vi "getState.vi"(8 "error in (no error)":errorcluster, 11 "Electrometer in":refnum<class "Electrometer.lvclass">) -> (0 "error out":errorcluster, 2 "State":T1, 3 "Electrometer out":refnum<class "Electrometer.lvclass">)   [LabVIEW 2016, in "Electrometer.lvclass"]
uses:
  Electrometer.lvclass
  internalState.ctl
  State/State.lvclass
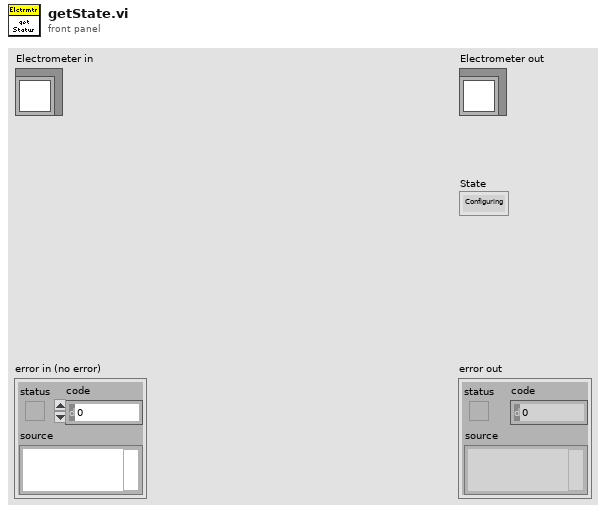
[diagram p1: front panel]
types:
  T1 = typedef "Electrometer.lvclass/internalState.ctl" = enum16{"Configuring", "Ready", "Reading"}
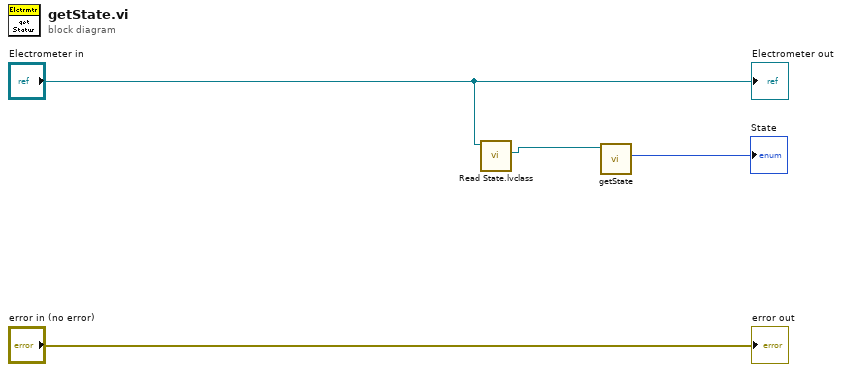
[diagram p0: block diagram]
diagram:
  n1 = call-dynamic "Read State.lvclass.vi"("Electrometer in"="Electrometer in") -> ("State.lvclass"=w2:refnum<class "State.lvclass">)  [unwired: 8 in, 2 out]
  n2 = call-dynamic "getState.vi"("State in"=w2) -> ("State"=→"State":T1)  [unwired: 8 in, 2 out]
  "error out" <- "error in (no error)"
  "Electrometer out" <- "Electrometer in"
